vi "FTW-ERR-ThrowImpossibleError.vi"(7 "Reason this error should never happen":string, 11 "error in":errorcluster) -> (15 "error out":errorcluster)   [LabVIEW 2014]
doc: "Toto, I've a feeling we're not in Kansas any more.... We must be over the rainbow!"
panel:
  # "Inputs"
  # "Outputs"
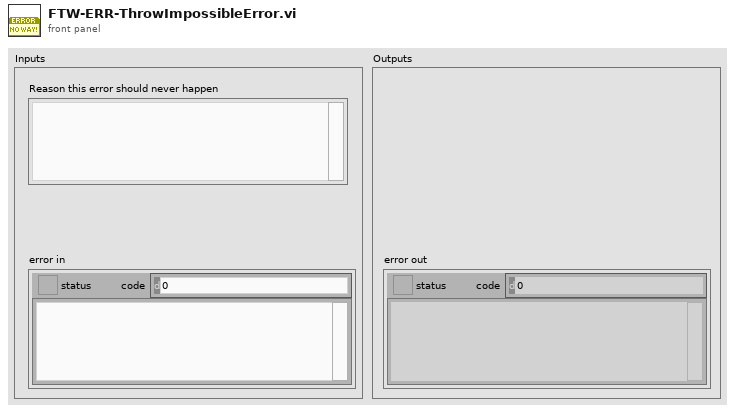
[diagram p1: front panel]
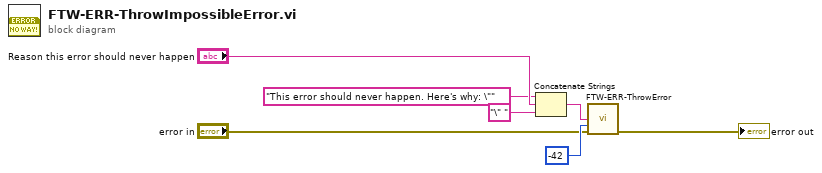
[diagram p0: block diagram]
diagram:
  n1 = Concatenate Strings("This error should never happen. Here's why: \"" ("string"), "Reason this error should never happen", "\" " ("string")) -> (w1:string)
  n2 = call "FTW-ERR-ThrowError.vi"("Error Message"=w1, "Error Code"=-42 ("code"), "error in"="error in") -> ("error out"=→"error out":errorcluster)  [unwired: 12 in]
